vi "N5765A_SetVoltageCurrent.vi"(6 "Current Limit (amps)":dbl format="%^.3e", 7 "Voltage Level":dbl format="%^.3e", 8 "error in (no error)":errorcluster, 11 "VISA resource name":refnum<visa-resource-name>) -> (0 "error out":errorcluster, 3 "VISA out":refnum<visa-resource-name>)   [LabVIEW 2015]
doc: "This VI will set the Voltage taking into acount the polarity and the Current of the Power Supply\n\nThe input is an array of setting to allow the user to set all or one channel on as many devices as required"
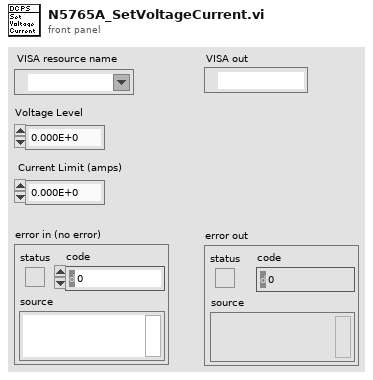
[diagram p1: front panel]
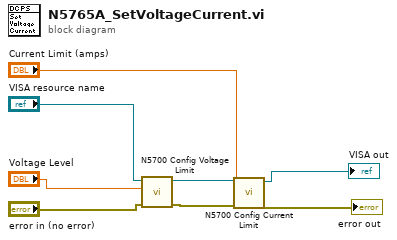
[diagram p0: block diagram]
diagram:
  n1 = call <instrlib>:"N5700 Config Voltage Limit.vi"("error"="error in (no error)", "Volt Limit"="Voltage Level", "VISA"="VISA resource name") -> ("error out"=w7:errorcluster, "VISA out"=w2:refnum<visa-resource-name>)  [unwired: 4 in]
  n2 = call <instrlib>:"N5700 Config Current Limit.vi"("error"=w7, "Current Limit"="Current Limit (amps)", "VISA"=w2) -> ("error out"=→"error out":errorcluster, "VISA out"=→"VISA out":refnum<visa-resource-name>)  [unwired: 4 in]
